vi "Толщиномер.vi"() -> ()   [LabVIEW 2016]
uses:
  <vilib>/Instr/_visa.llb/VISA Configure Serial Port (Instr).vi
  <vilib>/Platform/browser.llb/Open URL in Default Browser (string).vi
panel:
  in  "Process Stop Button":bool
  in  "Mail Button":bool
  in  "Paste Button":bool
  in  "Help Button":bool
  out "Ошибки 3":bool
  out "Режим отладки: 2":bool
  out "Ошибки 2":bool
  in  "Вкл. ScrollBar":bool
  in  "Цвет элементов:":u32(colorbox)=13027014
  in  "Цвет фона::":u32(colorbox)=14935011
  in  "Дата и время:":timestamp=timestamp(3752940422.3935633 s since 1904-01-01) format="%<%H:%M:%S\n%d/%m/%y>T"
  out "n:":dbl=1.0 format="%#_4f"
  in  "Показатель преломления:":dbl=1.5
  out "Пропускание T:":dbl
  out "Отражение R:":dbl
  out "a:":dbl format="%#_4g"
  out "Numeric":dbl
  out "Ответ МК:":string="Откл."
  out "Питание, В":dbl=3.28695
  in  "Яркость источника света":i32(knob)=255 scale=127.0..255.0
  in  "OK Button 5":bool
  out "Команда:":string="Откл."
  in  "Питание LED":bool
  in  "Скорость (бод)":dbl=115200.0
  in  "Порт ввода/вывода":refnum<visa-resource-name>="COM3"
  in  "Материал:":string="Титан"
  in  "Заметка:":string="Тестовое измерение"
  in  "Экспериментатор:":string="Студент"
  out "Толщина пленки:":dbl format="%#_4e"
  in  "OK Button 4":bool
  in  "OK Button 3":bool
  in  "Показатель поглощения:":dbl=100000.0 format="%#_6e"
  in  "Выбор материала пленки":T1(radio)
  in  "Показать значение тока с фотоприемника:":bool
  out "мкА":dbl
  out "Результат (код):":i32
  in  "OK Button 2":bool
  out "мкА":dbl
  out "Результат (код):":i32
  in  "OK Button":bool
  in  "Путь:":path=path "D:/Учебные материалы 3-4 курс/9 семестр/КТ/Лабы/mk/test1.txt"
  in  "Режим отладки:":bool
  in  "Включить перевод уровней АЦП в значения тока":bool
  out "Сигнал с фотоприемника":dbl(knob) scale=0.0..40.0
  # "Иземерения"
  # "->"
  # "->"
  # "Результаты"
  # "мкА"
  # "м"
  # "Сохранение результатов работы:"
  # "1/см"
  # "1/см"
  # "мкА"
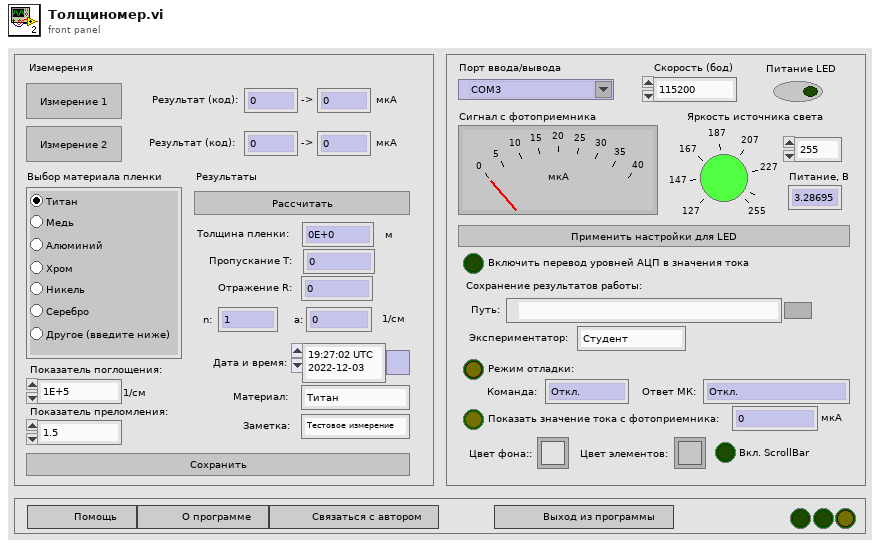
[diagram p1: front panel]
types:
  T1 = enum32{"Radio Selection 1", "Radio Selection 2", "Radio Selection 3", "Radio Selection 4", "Radio Selection 5", "Radio Selection 6", "Radio Selection 7"}
  T2 = cluster{"Цвет элементов:":u32, "Цвет элементов:":u32}
  T3 = cluster{"Цвет элементов:":u32, "Цвет элементов:":u32}[]
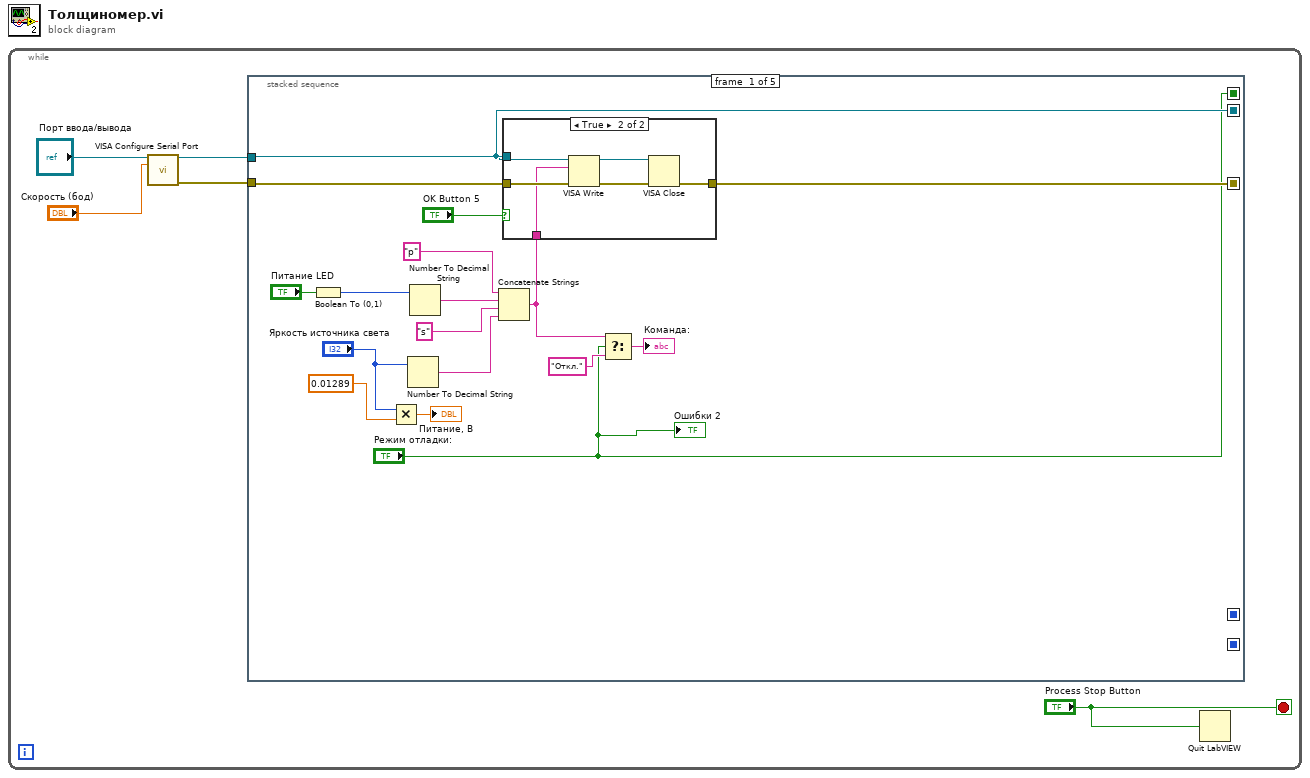
[diagram p0: block diagram]
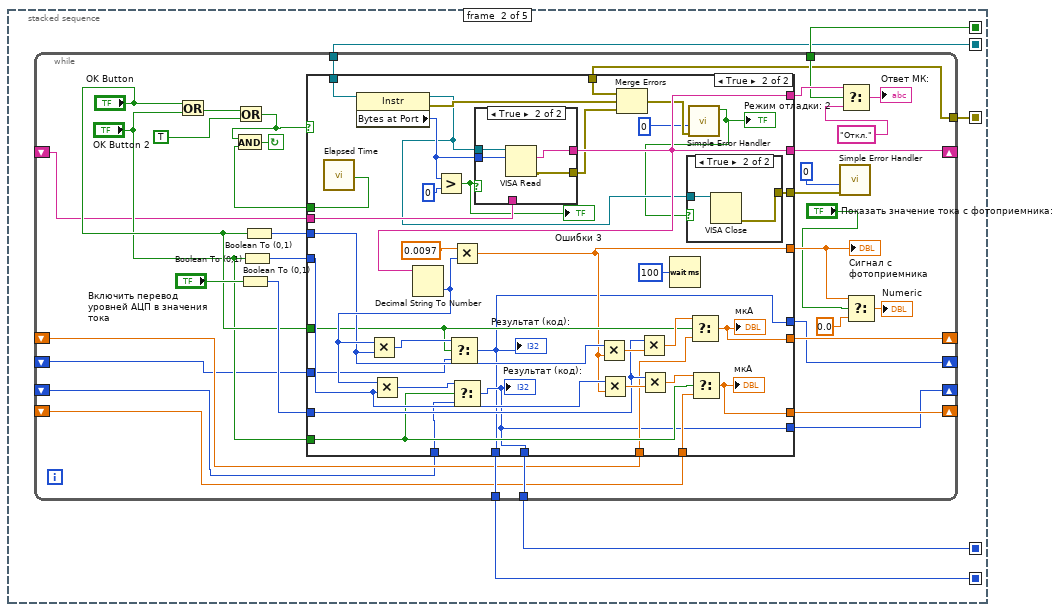
[diagram p3: hidden frame]
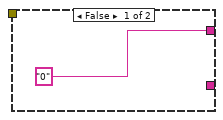
[diagram p4: hidden frame]
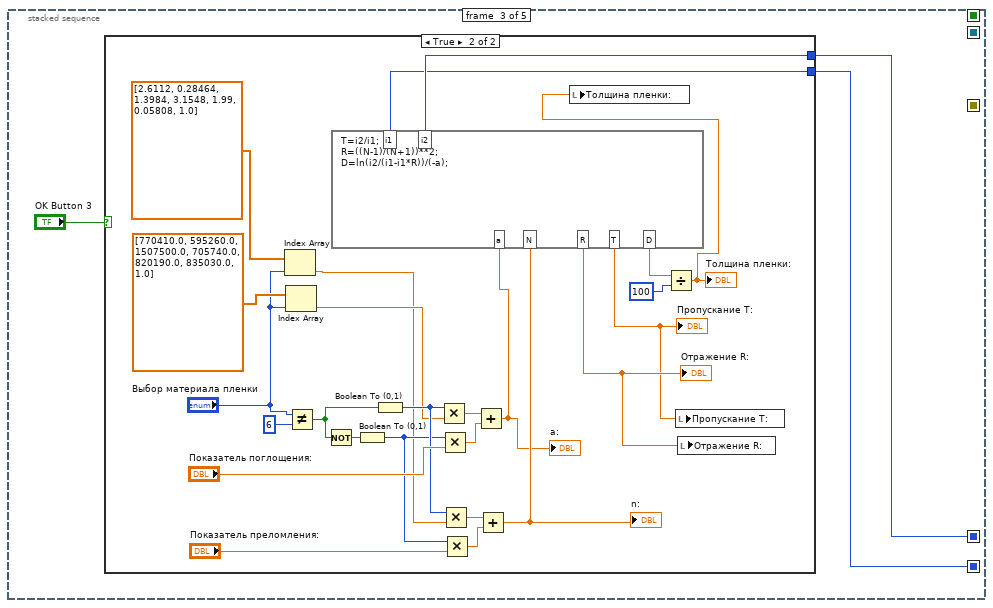
[diagram p7: hidden frame]
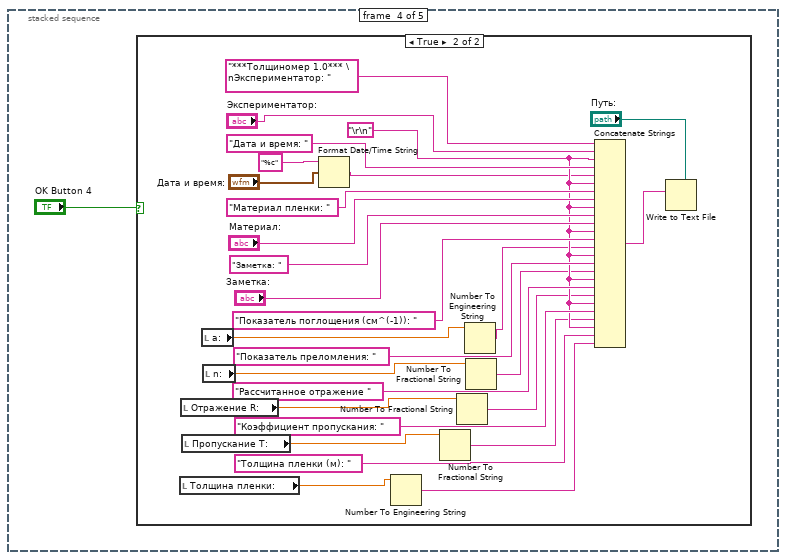
[diagram p9: hidden frame]
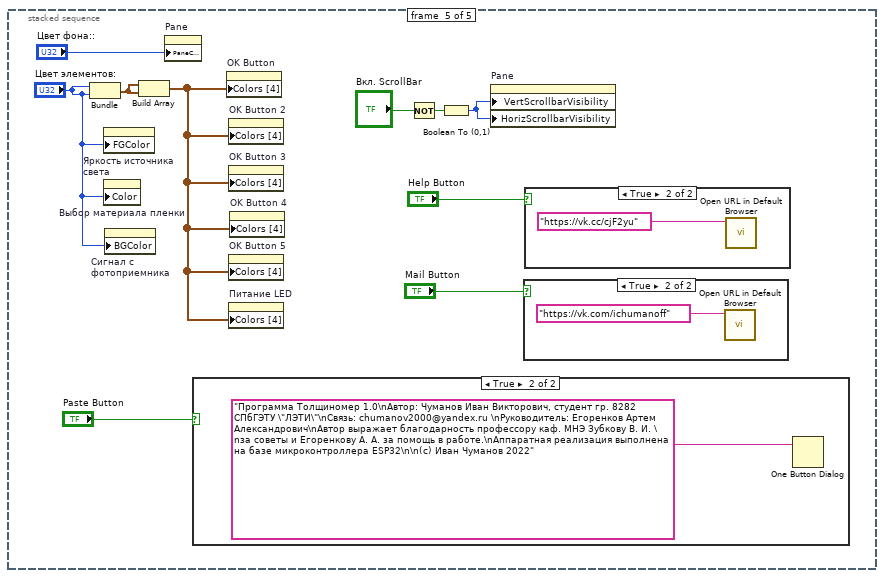
[diagram p11: hidden frame]
diagram:
  n1 = while {
    stop <- "Process Stop Button" stop-if-true
    n2 = call-poly "VISA Configure Serial Port"("VISA resource name"="Порт ввода/вывода", "baud rate (9600)"="Скорость (бод)") -> ("VISA resource name out"=w2:refnum<visa-resource-name>, "error out"=w3:errorcluster)  [unwired: 12 in]
    n3 = stacked-sequence {
      seq-local: [w8 _ _ _ _] -> [_ w30 _ _ _]
      seq-local: ["Режим отладки:" _ _ _ _] -> [_ w31 _ _ _]
      seq-local: [_ w33 _ _ _] -> [_ _ w116 _ _]
      seq-local: [_ w32 _ _ _] -> [_ _ w115 _ _]
      seq-local: [w7 _ _ _ _] -> [_ w29 _ _ _]
      tunnel: w3 -> [w9 _ _ _ _]
      tunnel: w2 -> [w8 _ _ _ _]
      frame #0 {
        n4 = Boolean To (0,1)(Boolean="Питание LED") -> (0, 1=w11:i16)
        n5 = Multiply(x="Яркость источника света", y=0.01289) -> (x*y=→"Питание, В":dbl)
        n6 = Number To Decimal String(number="Яркость источника света") -> (decimal integer string=w15:string)  [unwired: 1 in]
        n7 = Number To Decimal String(number=w11) -> (decimal integer string=w13:string)  [unwired: 1 in]
        n8 = Concatenate Strings("p", w13, "s", w15) -> (w20:string)
        n9 = case shown="True" "OK Button 5" {
          tunnel: w8 -> [_ w26]
          tunnel: w9 -> [_ w25]
          tunnel: w20 -> [_ w24]
          tunnel: [_ w23] -> w7
          frame False {
          }
          frame True {
            n10 = VISA Write(VISA resource name=w26, write buffer=w24, error in (no error)=w25) -> (VISA resource name out=w28:refnum<visa-resource-name>, error out=w27:errorcluster)  [unwired: 1 out]
            n11 = VISA Close(VISA resource name=w28, error in (no error)=w27) -> (error out=w23:errorcluster)
          }
        }
        n12 = Select(t=w20, s="Режим отладки:", f="Откл.") -> (s? t:f=→"Команда:":string)
        "Ошибки 2" <- "Режим отладки:"
      }
      frame #1 {
        n13 = while {
          tunnel: w30 -> [w68]
          tunnel: [w59] -> w33
          tunnel: [w58] -> w32
          tunnel: w31 -> [w52]
          shift-right: [w49] -> _
          shift-left: _ -> [w48]
          shift-right: [w43] -> _
          shift-left: _ -> [w42]
          shift-right: [w45] -> _
          shift-left: _ -> [w44]
          shift-right: [w47] -> _
          shift-left: _ -> [w46]
          shift-right: [w41] -> _
          shift-left: _ -> [w40]
          tunnel: w29 -> [w39]
          stop <- w66 continue-if-true
          n14 = Or(x="OK Button", y="OK Button 2") -> (x .or. y?=w35:bool)
          n15 = Or(x=w35, y=TRUE) -> (x .or. y?=w36:bool)
          n16 = Boolean To (0,1)(Boolean="Включить перевод уровней АЦП в значения тока") -> (0, 1=w64:i16)
          n17 = Boolean To (0,1)(Boolean="OK Button 2") -> (0, 1=w62:i16)
          n18 = Boolean To (0,1)(Boolean="OK Button") -> (0, 1=w63:i16)
          n19 = case shown="True" w36 {
            tunnel: ["0" w80] -> w55
            tunnel: w68 -> [_ w104]
            tunnel: [_ w103] -> w67
            tunnel: w64 -> [_ w98]
            tunnel: w63 -> [_ w96]
            tunnel: w62 -> [_ w95]
            tunnel: "OK Button" -> [_ w92]
            tunnel: "OK Button 2" -> [_ w90]
            tunnel: [_ w89] -> w53
            tunnel: [_ w82] -> w59
            tunnel: [_ w83] -> w58
            tunnel: w44 -> [_ w88]
            tunnel: [_ w87] -> w49
            tunnel: [_ w86] -> w47
            tunnel: w46 -> [_ w85]
            tunnel: w48 -> [_ w84]
            tunnel: [_ w83] -> w45
            tunnel: [_ w82] -> w43
            tunnel: w42 -> [_ w81]
            tunnel: [_ w80] -> w41
            tunnel: w40 -> [_ w79]
            tunnel: w39 -> [_ w74]
            tunnel: [_ w72] -> w38
            frame False {
            }
            frame True {
              n20 = call "Elapsed Time"() -> ("Time has Elapsed"=w103:bool)  [unwired: 12 in, 7 out]
              n21 = property class="Instr"(reference=w104) -> (reference out=w73:refnum<visa-resource-name>, error out=w77:errorcluster, "Bytes at Port"=w106:u32)  [unwired: 1 in]
              n22 = Greater?(x=w106, y=0) -> (0:w70:bool)
              "Ошибки 3" <- w70
              n23 = case shown="True" w70 {
                tunnel: w73 -> [_ w114]
                tunnel: w106 -> [_ w113]
                tunnel: [w110 w112] -> w80
                tunnel: [_ w111] -> w78
                tunnel: w79 -> [w110 _]
                frame False {
                }
                frame True {
                  n24 = VISA Read(VISA resource name=w114, byte count=w113) -> (read buffer=w112:string, error out=w111:errorcluster)  [unwired: 1 in, 2 out]
                }
              }
              n25 = Decimal String To Number(string=w80) -> (number=w99:i32)  [unwired: 2 in, 1 out]
              n26 = Multiply(x=w99, y=w96) -> (x*y=w93:i32)
              n27 = Multiply(x=w99, y=w95) -> (x*y=w91:i32)
              n28 = Select(t=w93, s=w92, f=w81) -> (s? t:f=w82:i32)
              "Результат (код):" <- w82
              n29 = Multiply(x=0.0097, y=w99) -> (x*y=w89:dbl)
              n30 = Select(t=w91, s=w90, f=w88) -> (s? t:f=w83:i32)
              "Результат (код):" <- w83
              n31 = Multiply(x=w96, y=w89) -> (x*y=w101:dbl)
              n32 = Multiply(x=w95, y=w89) -> (x*y=w102:dbl)
              n33 = Merge Errors(w74, w77, w78) -> (w76:errorcluster)
              n34 = Multiply(x=w98, y=w101) -> (x*y=w97:dbl)
              n35 = Multiply(x=w98, y=w102) -> (x*y=w94:dbl)
              n36 = Wait (ms)(milliseconds to wait=100) -> ()  [unwired: 1 out]
              n37 = call <vilib>:"Simple Error Handler.vi"("type of dialog (OK msg:1)"=0, "error in (no error)"=w76) -> ("error?"=w71:bool)  [unwired: 3 in, 4 out]
              "Режим отладки: 2" <- w71
              n38 = case shown="True" w71 {
                tunnel: w73 -> [_ w109]
                tunnel: [_ w108] -> w72
                frame False {
                }
                frame True {
                  n39 = VISA Close(VISA resource name=w109) -> (error out=w108:errorcluster)  [unwired: 1 in]
                }
              }
              n40 = Select(t=w97, s=w92, f=w84) -> (s? t:f=w87:dbl)
              "мкА" <- w87
              n41 = Select(t=w94, s=w90, f=w85) -> (s? t:f=w86:dbl)
              "мкА" <- w86
            }
          }
          "Сигнал с фотоприемника" <- w53
          n42 = And(x=w36, y=w67) -> (x .and. y?=w66:bool)
          n43 = call <vilib>:"Simple Error Handler.vi"("type of dialog (OK msg:1)"=0, "error in (no error)"=w38) -> ()  [unwired: 3 in, 5 out]
          n44 = Select(t=w55, s=w52, f="Откл.") -> (s? t:f=→"Ответ МК:":string)
          n45 = Select(t=w53, s="Показать значение тока с фотоприемника:", f=0.0) -> (s? t:f=→"Numeric":dbl)
        }
      }
      frame #2 {
        n46 = case shown="True" "OK Button 3" {
          tunnel: w116 -> [_ w119]
          tunnel: w115 -> [_ w120]
          frame False {
          }
          frame True {
            n47 = Index Array(array=dbl[] [2.6112, 0.28464, 1.3984, 3.1548, 1.99, 0.05808, 1.0], index="Выбор материала пленки") -> (element=w124:dbl)
            n48 = Index Array(array=dbl[] [770410.0, 595260.0, 1507500.0, 705740.0, 820190.0, 835030.0, 1.0], index="Выбор материала пленки") -> (element=w125:dbl)
            n49 = Not Equal?(x="Выбор материала пленки", y=6) -> (x != y?=w142:bool)
            n50 = Not(x=w142) -> (.not. x?=w141:bool)
            n51 = Boolean To (0,1)(Boolean=w141) -> (0, 1=w130:i16)
            n52 = Boolean To (0,1)(Boolean=w142) -> (0, 1=w131:i16)
            n53 = Multiply(x=w131, y=w125) -> (x*y=w138:dbl)
            n54 = Multiply(x=w130, y="Показатель поглощения:") -> (x*y=w139:dbl)
            n55 = Multiply(x=w131, y=w124) -> (x*y=w133:dbl)
            n56 = Multiply(x=w130, y="Показатель преломления:") -> (x*y=w132:dbl)
            n57 = Add(x=w138, y=w139) -> (x+y=w123:dbl)
            "a:" <- w123
            n58 = Add(x=w133, y=w132) -> (x+y=w128:dbl)
            "n:" <- w128
            n59 = formula code="T=i2/i1;\nR=((N-1)/(N+1))**2;\nD=ln(i2/(i1-i1*R))/(-a);"("i1"=w119, "i2"=w120, "a"=w123, "N"=w128) -> ("T"=w118:dbl, "R"=w122:dbl, "D"=w127:dbl)
            "Пропускание T:" <- w118
            "Отражение R:" <- w122
            n60 = Divide(x=w127, y=100) -> (x/y=w121:dbl)
            "Толщина пленки:" <- w121
            n61 = local write "Толщина пленки:"(w121) -> ()
            n62 = local write "Пропускание T:"(w118) -> ()
            n63 = local write "Отражение R:"(w122) -> ()
          }
        }
      }
      frame #3 {
        n64 = case shown="True" "OK Button 4" {
          frame False {
          }
          frame True {
            w158 = "\r\n"
            n65 = local read "Толщина пленки:"() -> (w152:dbl)
            n66 = local read "Отражение R:"() -> (w149:dbl)
            n67 = local read "Пропускание T:"() -> (w150:dbl)
            n68 = local read "a:"() -> (w147:dbl)
            n69 = local read "n:"() -> (w144:dbl)
            n70 = Format Date/Time String(time format string (%c)="%c", seconds (now)="Дата и время:") -> (date/time string=w156:string)  [unwired: 1 in]
            n71 = Number To Engineering String(4:w152) -> (0:w153:string)  [unwired: 3 in]
            n72 = Number To Fractional String(number=w150) -> (F-format string=w151:string)  [unwired: 3 in]
            n73 = Number To Fractional String(number=w149) -> (F-format string=w148:string)  [unwired: 3 in]
            n74 = Number To Engineering String(4:w147) -> (0:w146:string)  [unwired: 3 in]
            n75 = Number To Fractional String(number=w144) -> (F-format string=w145:string)  [unwired: 3 in]
            n76 = Concatenate Strings("***Толщиномер 1.0*** \nЭкспериментатор: ", "Экспериментатор:", w158, "Дата и время: ", w156, w158, "Материал пленки: ", "Материал:", w158, "Заметка: ", "Заметка:", w158, "Показатель поглощения (см^(-1)): ", w146, w158, "Показатель преломления: ", w145, w158, "Рассчитанное отражение ", w148, w158, "Коэффициент пропускания: ", w151, w158, "Толщина пленки (м): ", w153) -> (w169:string)
            n77 = Write to Text File(file (use dialog)="Путь:", text=w169) -> ()  [unwired: 2 in, 3 out]
          }
        }
      }
      frame #4 {
        n78 = Bundle("Цвет элементов:"="Цвет элементов:", "Цвет элементов:"="Цвет элементов:") -> (w176:T2)  [unwired: 1 in]
        n79 = property on="Яркость источника света" class="Knob (strict)"("FGColor"="Цвет элементов:") -> ()  [unwired: 2 in, 2 out]
        n80 = property on="Выбор материала пленки" class="RadioBtnsControl (strict)"("Color"="Цвет элементов:") -> ()  [unwired: 2 in, 2 out]
        n81 = property on="Сигнал с фотоприемника" class="Knob (strict)"("BGColor"="Цвет элементов:") -> ()  [unwired: 2 in, 2 out]
        n82 = Build Array(w176, w176) -> (w177:T3)
        n83 = property on="Pane" class="Pane"("PaneColor"="Цвет фона::") -> ()  [unwired: 2 in, 2 out]
        n84 = case shown="True" "Paste Button" {
          frame False {
          }
          frame True {
            n85 = One Button Dialog(message="Программа Толщиномер 1.0\nАвтор: Чуманов Иван Викторович, студент гр. 8282 СПбГЭТУ \"ЛЭТИ\"\nСвязь: chumanov2000@yandex.ru \nРуководитель: Егоренков Артем Александрович\nАвтор выражает благодарность профессору каф. МНЭ Зубкову В. И. \nза советы и Егоренкову А. А. за помощь в работе.\nАппаратная реализация выполнена на базе микроконтроллера ESP32\n\n(с) Иван Чуманов 2022") -> ()  [unwired: 1 in, 1 out]
          }
        }
        n86 = property on="OK Button" class="Bool"("Colors [4]"=w177) -> ()  [unwired: 2 in, 2 out]
        n87 = property on="OK Button 2" class="Bool"("Colors [4]"=w177) -> ()  [unwired: 2 in, 2 out]
        n88 = property on="OK Button 3" class="Bool"("Colors [4]"=w177) -> ()  [unwired: 2 in, 2 out]
        n89 = property on="OK Button 5" class="Bool"("Colors [4]"=w177) -> ()  [unwired: 2 in, 2 out]
        n90 = property on="Питание LED" class="Bool (strict)"("Colors [4]"=w177) -> ()  [unwired: 2 in, 2 out]
        n91 = property on="OK Button 4" class="Bool"("Colors [4]"=w177) -> ()  [unwired: 2 in, 2 out]
        n92 = Not(x="Вкл. ScrollBar") -> (.not. x?=w180:bool)
        n93 = Boolean To (0,1)(Boolean=w180) -> (0, 1=w179:i16)
        n94 = property on="Pane" class="Pane"("VertScrollbarVisibility"=w179, "HorizScrollbarVisibility"=w179) -> ()  [unwired: 2 in, 2 out]
        n95 = case shown="True" "Mail Button" {
          frame False {
          }
          frame True {
            n96 = call-poly <vilib>:"Open URL in Default Browser.vi"("URL"="https://vk.com/ichumanoff") -> ()  [unwired: 5 in, 2 out]
          }
        }
        n97 = case shown="True" "Help Button" {
          frame False {
          }
          frame True {
            n98 = call-poly <vilib>:"Open URL in Default Browser.vi"("URL"="https://vk.cc/cjF2yu") -> ()  [unwired: 5 in, 2 out]
          }
        }
      }
    }
    n99 = Quit LabVIEW(quit? (T)="Process Stop Button") -> ()
  }
